vi "test_dll.vi"() -> ()   [LabVIEW 2015]
uses:
  C:/Users/MAHA/Desktop/delele/bin/Debug/delele.dll
panel:
  out "return type":i32
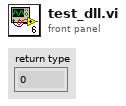
[diagram p1: front panel]
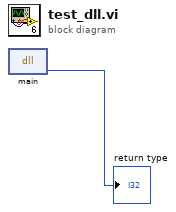
[diagram p0: block diagram]
diagram:
  n1 = dll-call lib="C:/Users/MAHA/Desktop/delele/bin/Debug/delele.dll" fn="main"() -> ("return type"=→"return type":i32)  [unwired: 3 in, 2 out]
